vi "Read Input Data.vi"(11 "TestDataLog in":refnum<class "TestDataLog.lvclass">) -> (2 "Input Data":T1={"Temperature Measured"=275.15, "ADCs"={"Ch0"=0, "Ch1"=0, "Ch2"=0, "Ch3"=0, "Ch4"=0}} {"Temperature Measured" min=271.15 max=275.15 format="%.1f"}, 3 "TestDataLog out":refnum<class "TestDataLog.lvclass">)   [LabVIEW 2013, in "TestDataLog.lvclass"]
uses:
  TestDataLog.lvclass
  Typedefs/InputData.ctl
  <userlib>/Common/ILC/Typedefs/ADCs.ctl
  TestDataLog.lvclass/TestDataLog.ctl
  <userlib>/Common/ILC/Typedefs/ILCTypedefs.lvlib
  Typedefs/AITDTTypedefs.lvlib
panel:
  # "ADCs"
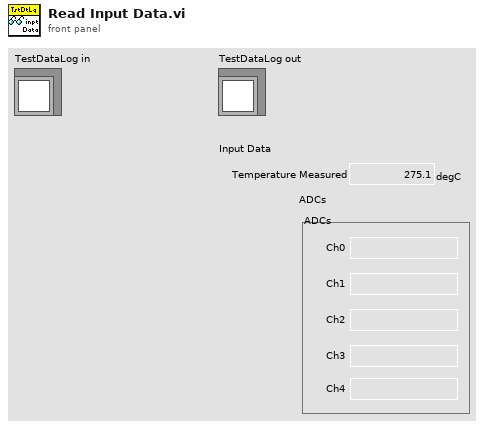
[diagram p1: front panel]
types:
  T1 = typedef "AITDTTypedefs.lvlib/InputData.ctl" = cluster{"Temperature Measured":dbl[unit], "ADCs":T2}
  T2 = typedef "ILCCommon.lvlib/ILCTypedefs.lvlib/ADCs.ctl" = cluster{"Ch0":i32, "Ch1":i32, "Ch2":i32, "Ch3":i32, "Ch4":i32}
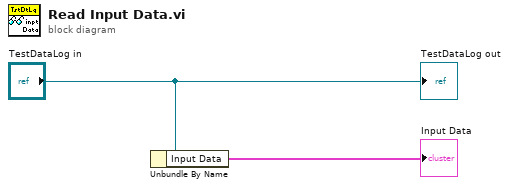
[diagram p0: block diagram]
diagram:
  n1 = Unbundle By Name("TestDataLog in") -> ("Input Data"=→"Input Data":T1)
  "TestDataLog out" <- "TestDataLog in"
